vi "Invert u32.vi"(10 "In (u16)":u32) -> (2 "Out (u16)":u32)   [LabVIEW 2015]
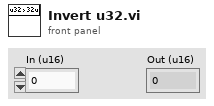
[diagram p1: front panel]
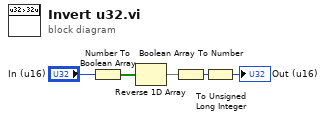
[diagram p0: block diagram]
diagram:
  n1 = Number To Boolean Array(number="In (u16)") -> (Boolean array=w5:bool[])
  n2 = Reverse 1D Array(array=w5) -> (reversed array=w4:bool[])
  n3 = Boolean Array To Number(Boolean array=w4) -> (number=w3:u32)
  n4 = To Unsigned Long Integer(number=w3) -> (unsigned 32bit integer=→"Out (u16)":u32)
